vi "AD7747_Init.vi"(4 "FPGA":T1, 8 "error in":errorcluster) -> (0 "error out":errorcluster)   [LabVIEW 2012]
uses:
  Type Defs/WSVCAP SHL FPGA Enum.ctl
panel:
  # "Initialize AD7747 for Capacitance Measurement Mode"
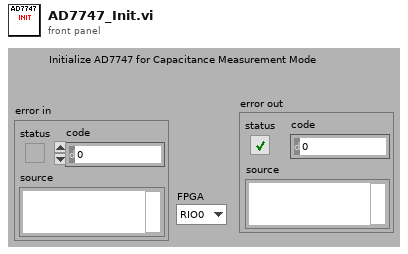
[diagram p1: front panel]
types:
  T1 = typedef "WSVCAP SHL FPGA Enum.ctl" = enum16{"RIO0", "RIO1"}
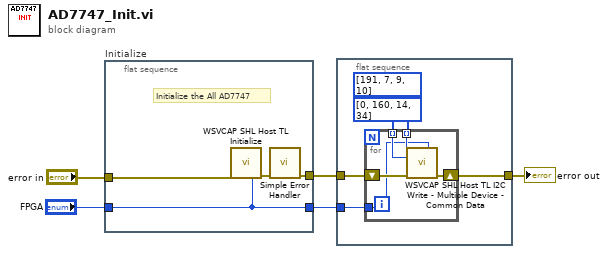
[diagram p0: block diagram]
diagram:
  n1 = flat-sequence "Initialize" {
    tunnel: "error in" -> [w7]
    tunnel: [w8] -> w4
    tunnel: "FPGA" -> [w6]
    tunnel: [w6] -> w1
    frame #0 {
      # "Initialize the All AD7747"
      n2 = call "WSVCAP SHL Host TL Initialize.vi"("error in"=w7, "FPGA"=w6) -> ("error out"=w9:errorcluster)  [unwired: 12 in, 1 out]
      n3 = call <vilib>:"Simple Error Handler.vi"("error in (no error)"=w9) -> ("error out"=w8:errorcluster)  [unwired: 4 in, 4 out]
    }
  }
  n4 = flat-sequence {
    tunnel: w4 -> [w12]
    tunnel: [w11] -> w3
    tunnel: w1 -> [w10]
    frame #0 {
      n5 = for {
        tunnel: u8[] [191, 7, 9, 10] -> [w19] mode=indexing
        tunnel: u8[] [0, 160, 14, 34] -> [w18] mode=indexing
        shift-right: [w17] -> w11
        shift-left: w12 -> [w16]
        tunnel: w10 -> [w15]
        n6 = call "WSVCAP SHL Host TL I2C Write - Multiple Device - Common Data.vi"("Sub Address"=w19, "FPGA"=w15, "Data Out [U8]"=w18, "error in"=w16) -> ("error out"=w17:errorcluster)  [unwired: 11 in]
      }
    }
  }
  "error out" <- w3
